vi "writeROIXML.vi"(8 "error in (no error)":errorcluster, 11 "ImageStreamViewer in":refnum<class "ImageStreamViewer.lvclass">) -> (0 "error out":errorcluster, 3 "ImageStreamViewer out":refnum<class "ImageStreamViewer.lvclass">)   [LabVIEW 2009, in "Views.lvlib" / "Camera.lvlib" / "ImageStreamViewer.lvclass"]
uses:
  ImageStreamViewer.lvclass
  ImageStreamViewer.lvclass/ImageStreamViewer.ctl
  Tools/NativeXML/NativeXML.lvclass
  Tools/Filing/FileSystem/FileSystem.lvclass
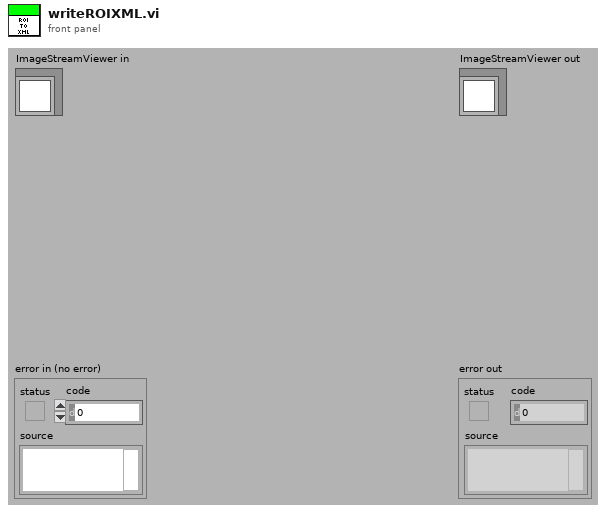
[diagram p1: front panel]
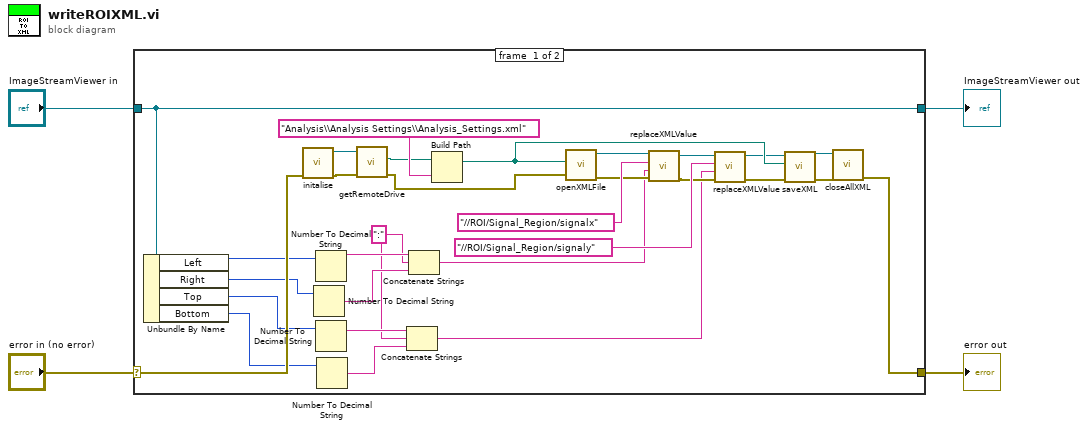
[diagram p0: block diagram]
diagram:
  n1 = case shown="No Error" "error in (no error)" {
    selector: "error in (no error)" -> [w22 w36]
    tunnel: [w30 w36] -> w3
    tunnel: [w23 w35] -> w1
    tunnel: "ImageStreamViewer in" -> [w23 w35]
    frame #0 {
      w9 = ":"
      n2 = Unbundle By Name(w23) -> ("Left"=w16:i32, "Right"=w15:i32, "Top"=w14:i32, "Bottom"=w13:i32)
      n3 = call "initalise.vi"("error in (no error)"=w22) -> ("error out"=w28:errorcluster, "FileSystem out"=w27:refnum<class "FileSystem.lvclass">)  [unwired: 9 in]
      n4 = Number To Decimal String(number=w15) -> (decimal integer string=w11:string)  [unwired: 1 in]
      n5 = Number To Decimal String(number=w16) -> (decimal integer string=w12:string)  [unwired: 1 in]
      n6 = Number To Decimal String(number=w14) -> (decimal integer string=w10:string)  [unwired: 1 in]
      n7 = Number To Decimal String(number=w13) -> (decimal integer string=w8:string)  [unwired: 1 in]
      n8 = call "getRemoteDrive.vi"("error in (no error)"=w28, "FileSystem in"=w27) -> ("error out"=w21:errorcluster, "RemoteDrive"=w25:path)  [unwired: 7 in, 1 out]
      n9 = Concatenate Strings(w10, w9, w8) -> (w5:string)
      n10 = Concatenate Strings(w12, w9, w11) -> (w7:string)
      n11 = Build Path(base path=w25, name or relative path="Analysis\\Analysis Settings\\Analysis_Settings.xml") -> (appended path=w24:path)
      n12 = call "openXMLFile.vi"("error in (no error)"=w21, "Path"=w24) -> ("error out"=w29:errorcluster, "NativeXML out"=w31:refnum<class "NativeXML.lvclass">)  [unwired: 8 in]
      n13 = call "replaceXMLValue.vi"("error in (no error)"=w29, "value"=w7, "replace in"="//ROI/Signal_Region/signalx", "NativeXML in"=w31) -> ("error out"=w6:errorcluster, "NativeXML out"=w20:refnum<class "NativeXML.lvclass">)  [unwired: 6 in]
      n14 = call "replaceXMLValue.vi"("error in (no error)"=w6, "value"=w5, "replace in"="//ROI/Signal_Region/signaly", "NativeXML in"=w20) -> ("error out"=w18:errorcluster, "NativeXML out"=w19:refnum<class "NativeXML.lvclass">)  [unwired: 6 in]
      n15 = call "saveXML.vi"("error in (no error)"=w18, "Path"=w24, "NativeXML in"=w19) -> ("error out"=w34:errorcluster, "NativeXML out"=w33:refnum<class "NativeXML.lvclass">)  [unwired: 7 in]
      n16 = call "closeAllXML.vi"("error in (no error)"=w34, "NativeXML in"=w33) -> ("error out"=w30:errorcluster)  [unwired: 9 in]
    }
    frame #1 {
    }
  }
  "error out" <- w3
  "ImageStreamViewer out" <- w1
